vi "example.vi"() -> ()   [LabVIEW 2018]
uses:
  cat.lvclass
  D:/learning/animal.lvclass
  dog/dog.lvclass
  animal.lvclass
panel:
  in  "组合框":string(combo)
  in  "停止":bool
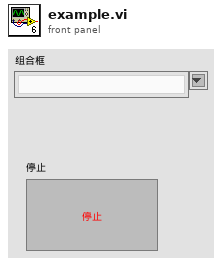
[diagram p1: front panel]
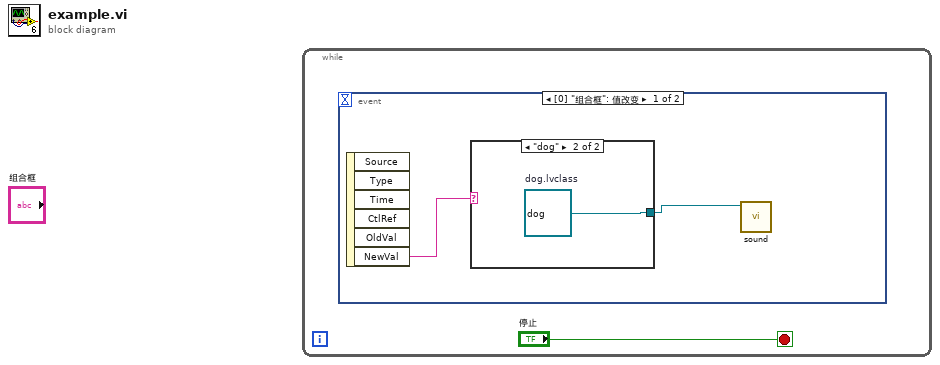
[diagram p0: block diagram]
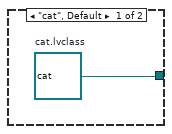
[diagram p2: hidden frame]
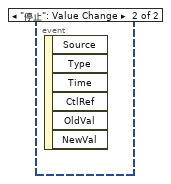
[diagram p3: hidden frame]
diagram:
  n1 = while {
    stop <- "停止" stop-if-true
    n2 = event shown="[0] \"组合框\": 值改变" {
      selector: _ -> [_ _]
      dyn-events: _ -> [_ _]
      timeout: _ -> [_ _]
      event "组合框": Value Change {
        n3 = event-data() -> ("NewVal"=w3:string)  [unwired: 1 in, 5 out]
        n4 = case shown="\"dog\"" w3 {
          tunnel: [w4 w5] -> w2
          frame "cat", Default {
            w4 = refnum<class "cat.lvclass"> refnum  # cat.lvclass
          }
          frame "dog" {
            w5 = refnum<class "dog.lvclass"> refnum  # dog.lvclass
          }
        }
        n5 = call-dynamic "sound.vi"("animal 输入"=w2) -> ()  [unwired: 9 in, 2 out]
      }
      event "停止": Value Change {
        n6 = event-data() -> ()  [unwired: 1 in, 6 out]
      }
    }
  }
